vi "Stop.vi"(8 "error in (no error)":errorcluster, 11 "KUKA youBot Wheel Motor in":refnum<class "NI_Robotics_KUKA youBot Wheel Motor.lvclass">) -> (0 "error out":errorcluster, 3 "KUKA youBot Wheel Motor out":refnum<class "NI_Robotics_KUKA youBot Wheel Motor.lvclass">)   [LabVIEW 2017, in "NI_Robotics_KUKA youBot Host.lvlib" / "NI_Robotics_KUKA youBot Wheel Motor.lvclass"]
uses:
  <vilib>/robotics/KUKA youBot/Motor/Wheel Motor/NI_Robotics_KUKA youBot Wheel Motor.lvclass
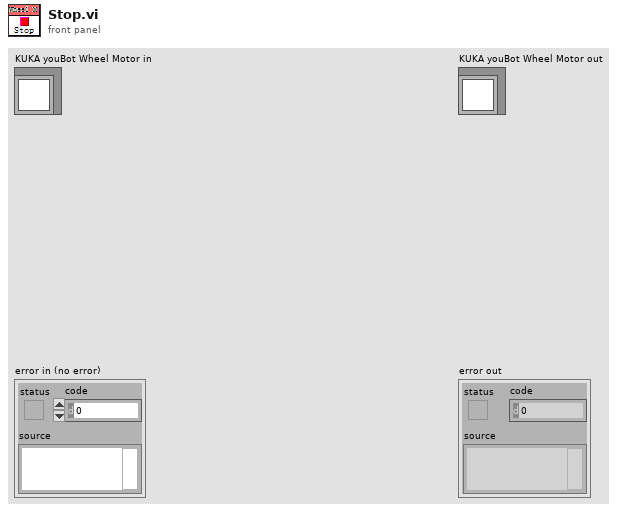
[diagram p1: front panel]
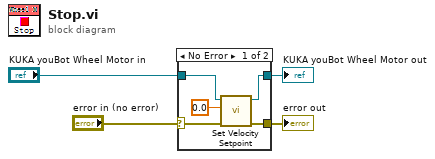
[diagram p0: block diagram]
diagram:
  n1 = case shown="No Error" "error in (no error)" {
    selector: "error in (no error)" -> [w6 w11]
    tunnel: [w5 w11] -> w3
    tunnel: [w8 w10] -> w1
    tunnel: "KUKA youBot Wheel Motor in" -> [w9 w10]
    frame No Error {
      n2 = call-dynamic "Set Velocity Setpoint.vi"("error in (no error)"=w6, "CCW velocity (rad/s)"=0.0, "KUKA youBot wheel motor in"=w9) -> ("error out"=w5:errorcluster, "KUKA youBot wheel motor out"=w8:refnum<class "NI_Robotics_KUKA youBot Wheel Motor.lvclass">)  [unwired: 7 in]
    }
    frame Error {
    }
  }
  "error out" <- w3
  "KUKA youBot Wheel Motor out" <- w1
